vi "Calculate_Obstace_Coordinates(SubVI).vi"(7 "Current_Position_in":T1, 8 "error in (no error)":errorcluster, 9 "SensorPos":dbl=0.172 format="%#_13g", 10 "SensorAngle":dbl, 11 "ObsDistance":dbl) -> (0 "error out":errorcluster, 1 "detected?":bool, 2 "Y_obs":dbl, 3 "X_obs":dbl)   [LabVIEW 2017]
uses:
  Ctl/Current_Position.ctl
  <vilib>/Analysis/coordinate.llb/Wrap Angle (scalar).vi
  <vilib>/Analysis/NI_AAL_Angle.lvlib
panel:
  out "AngleOfObs":dbl
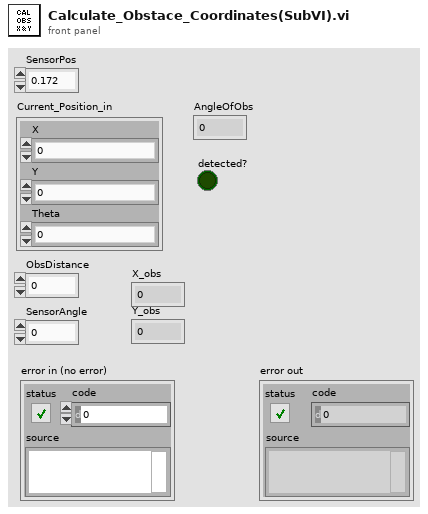
[diagram p1: front panel]
types:
  T1 = typedef "Current_Position.ctl" = cluster{"X":dbl, "Y":dbl, "Theta":dbl}
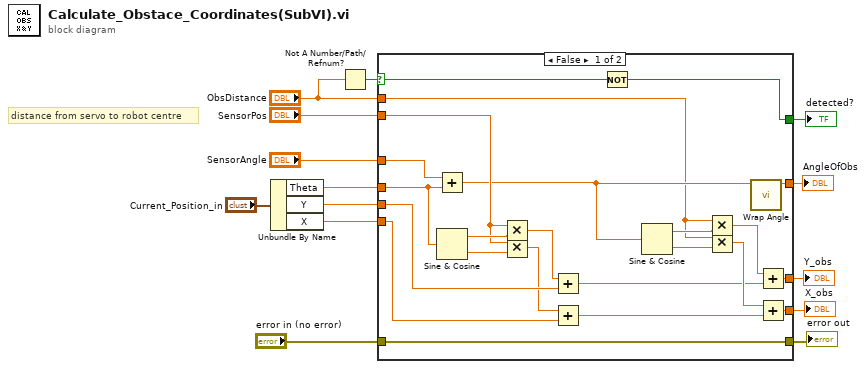
[diagram p0: block diagram]
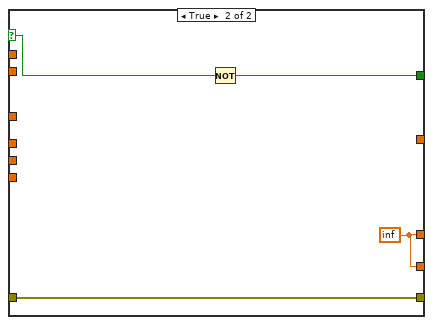
[diagram p2: hidden frame]
diagram:
  # "distance from servo to robot centre"
  n1 = Unbundle By Name("Current_Position_in") -> ("Theta"=w8:dbl, "Y"=w11:dbl, "X"=w10:dbl)
  n2 = Not A Number/Path/Refnum?(number/path/refnum="ObsDistance") -> (NaN/Path/Refnum?=w2:bool)
  n3 = case shown="False" w2 {
    selector: w2 -> [w17 w41]
    tunnel: [w37 _] -> w14
    tunnel: "SensorAngle" -> [w36 _]
    tunnel: w11 -> [w35 _]
    tunnel: w10 -> [w34 _]
    tunnel: "SensorPos" -> [w31 _]
    tunnel: w8 -> [w28 _]
    tunnel: "ObsDistance" -> [w20 _]
    tunnel: [w19 w38] -> w7
    tunnel: [w18 w38] -> w6
    tunnel: [w15 w39] -> w5
    tunnel: "error in (no error)" -> [w16 w40]
    tunnel: [w16 w40] -> w3
    frame False {
      n4 = Add(x=w36, y=w28) -> (x+y=w21:dbl)
      n5 = Sine & Cosine(0:w28) -> (1:w33:dbl, 2:w32:dbl)
      n6 = Multiply(x=w31, y=w33) -> (x*y=w30:dbl)
      n7 = Multiply(x=w31, y=w32) -> (x*y=w29:dbl)
      n8 = Add(x=w30, y=w35) -> (x+y=w22:dbl)
      n9 = Add(x=w29, y=w34) -> (x+y=w23:dbl)
      n10 = Not(x=w17) -> (.not. x?=w15:bool)
      n11 = Sine & Cosine(0:w21) -> (1:w27:dbl, 2:w26:dbl)
      n12 = Multiply(x=w20, y=w27) -> (x*y=w25:dbl)
      n13 = Multiply(x=w20, y=w26) -> (x*y=w24:dbl)
      n14 = call-poly <vilib>:"Wrap Angle.vi"("angle in"=w21) -> ("angle out"=w37:dbl)  [unwired: 9 in, 1 out]
      n15 = Add(x=w25, y=w22) -> (x+y=w19:dbl)
      n16 = Add(x=w24, y=w23) -> (x+y=w18:dbl)
    }
    frame True {
      w38 = inf
      n17 = Not(x=w41) -> (.not. x?=w39:bool)
    }
  }
  "AngleOfObs" <- w14
  "Y_obs" <- w7
  "X_obs" <- w6
  "error out" <- w3
  "detected?" <- w5
